vi "get average tour finding speed.vi"(1 "time spent running (seconds)":dbl format="%.3f", 2 "total no. of tours found":u64) -> (0 "avg. tour finding speed (tours/second)":string)   [LabVIEW 2020, in "main.lvlib"]
doc: "Blank VI with error handling."
uses:
  main.lvlib
  PTRL/string/string.lvlib
panel:
  # "Development\ncontrols/indicators useful for development and testing, but which are not outputs of the VI"
  # "Input\nInputs to the VI"
  # "Output\nOutputs of the VI"
  # "Description\n\nBlank VI with error handling case. \n\nSummarize the use of this VI in this space."
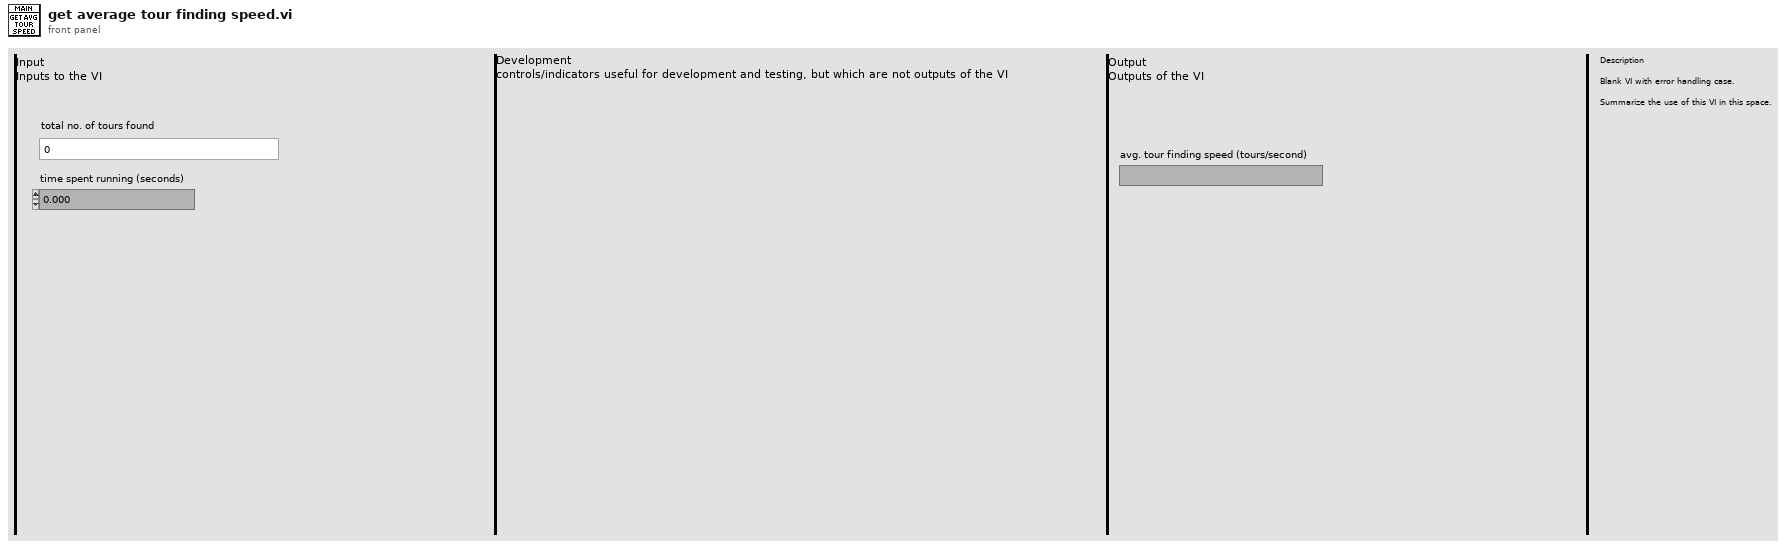
[diagram p1: front panel]
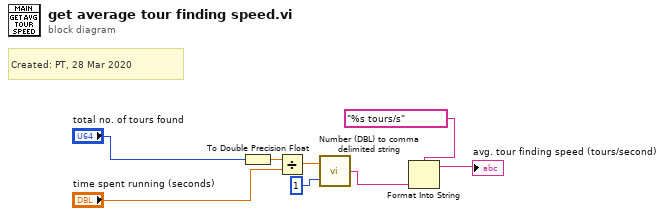
[diagram p0: block diagram]
diagram:
  # "Created: PT, 28 Mar 2020"
  n1 = To Double Precision Float(number="total no. of tours found") -> (double precision float=w8:dbl)
  n2 = Divide(x=w8, y="time spent running (seconds)") -> (x/y=w7:dbl)
  n3 = call "Number (DBL) to comma delimited string.vi"("precision (no. of decimals)"=i16 1, "Number"=w7) -> ("Comma delimited string"=w2:string)
  n4 = Format Into String(format string="%s tours/s", w2) -> (resulting string=→"avg. tour finding speed (tours/second)":string)  [unwired: 2 in, 1 out]
